vi "main.vi"() -> ()   [LabVIEW 2024]
uses:
  controls/#typedef_program_data_soundDB.ctl
  <vilib>/Utility/miscctls.llb/LVPoint32TypeDef.ctl
  controls/#typedef_program_states_soundDB.ctl
panel:
  out "error out":errorcluster
  in  "error in (no error)":errorcluster
  in  "Cluster":T1={"Sound intensity [dB]"=0, "Sound intensity: MIN"=0.0, "Sound intensity: MAX"=230.0, "Char array"=[], "Point32"={"Horizontal"=0, "Vertical"=0}, "drag?"=FALSE} {"Sound intensity [dB]" scale=0.0..100.0}
  out "To be moved":string
  in  "Sound intensity: MAX":dbl=230.0
  in  "Sound intensity: MIN":dbl
  out "Limit exceeded?":bool
  in  "Stop Button":bool
  in  "Sound intensity [dB]":u8(slide) scale=0.0..100.0
  # "85 dB"
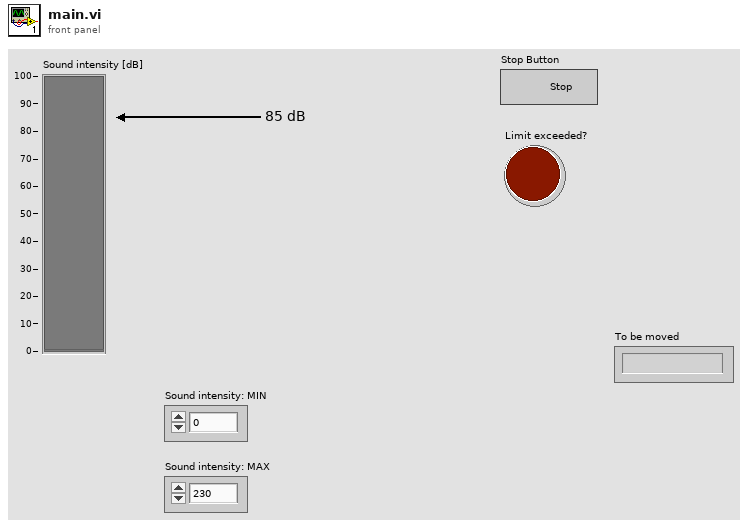
[diagram p1: front panel]
types:
  T1 = typedef "#typedef_program_data_soundDB.ctl" = cluster{"Sound intensity [dB]":u8, "Sound intensity: MIN":dbl, "Sound intensity: MAX":dbl, "Char array":i16[], "Point32":T2, "drag?":bool}
  T2 = typedef "LVPoint32TypeDef.ctl" = cluster{"Horizontal":i32, "Vertical":i32}
  T3 = typedef "#typedef_program_states_soundDB.ctl" = enum16{"application error", "init", "idle", "move", "Limit exceeded", "exit"}
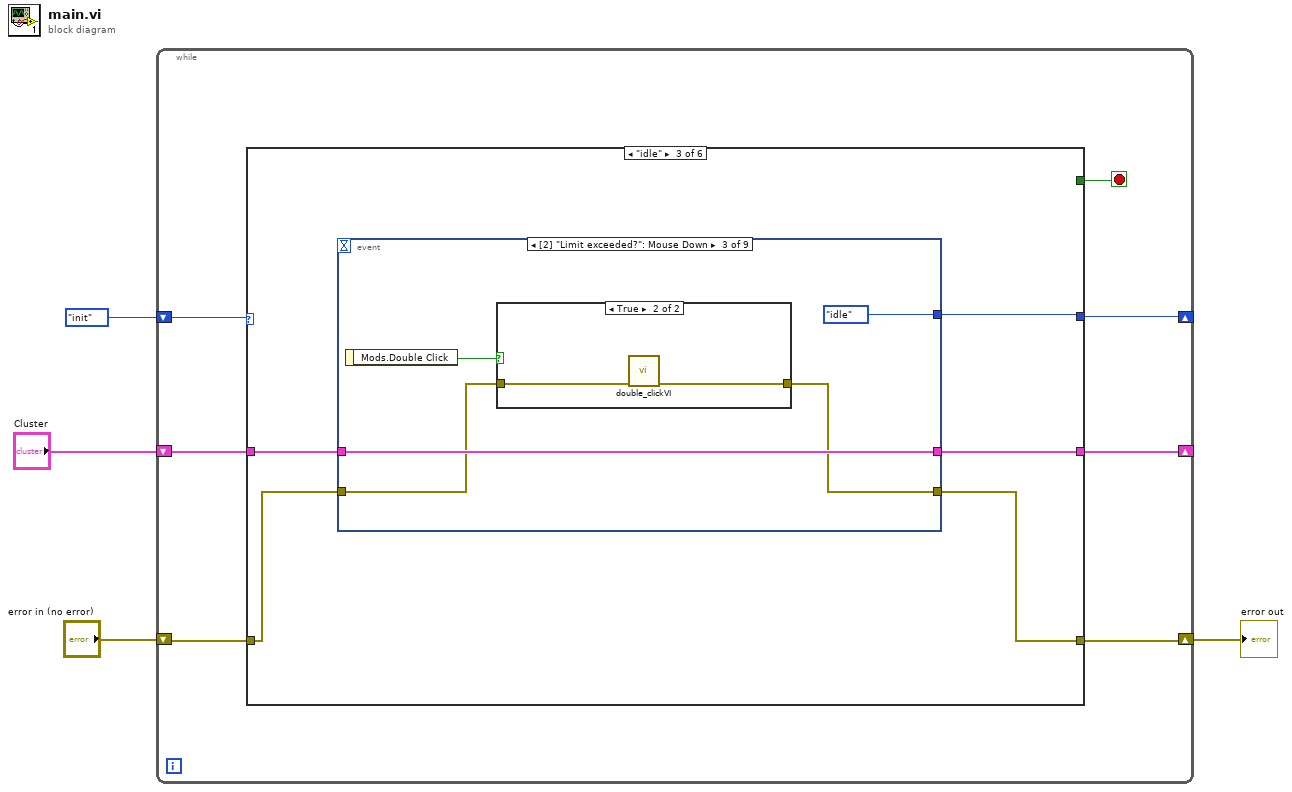
[diagram p0: block diagram]
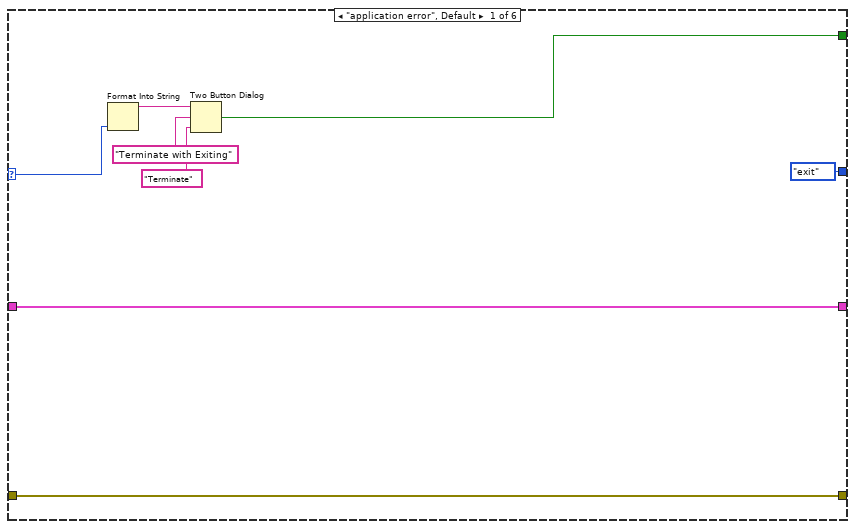
[diagram p2: hidden frame]
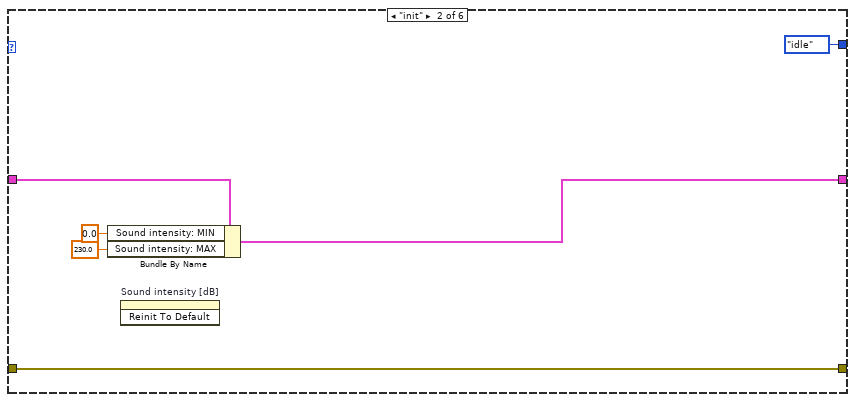
[diagram p3: hidden frame]
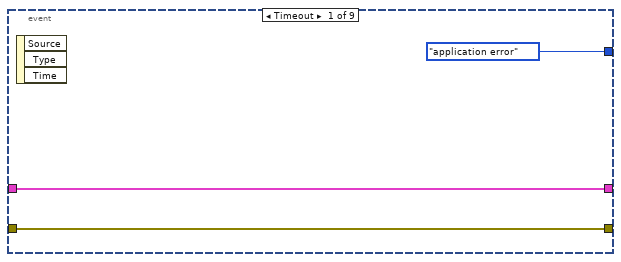
[diagram p4: hidden frame]
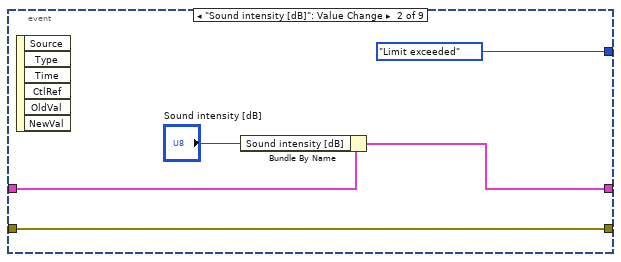
[diagram p5: hidden frame]
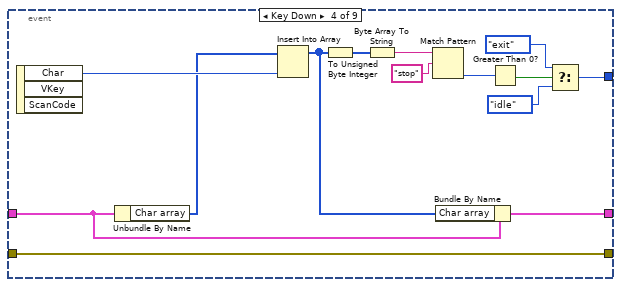
[diagram p7: hidden frame]
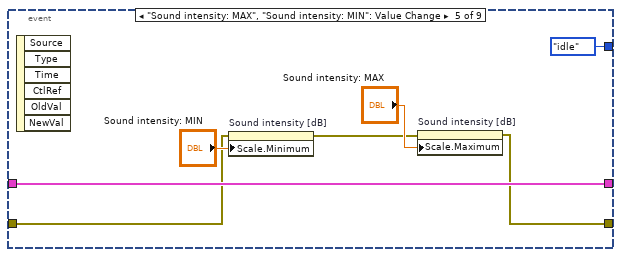
[diagram p8: hidden frame]
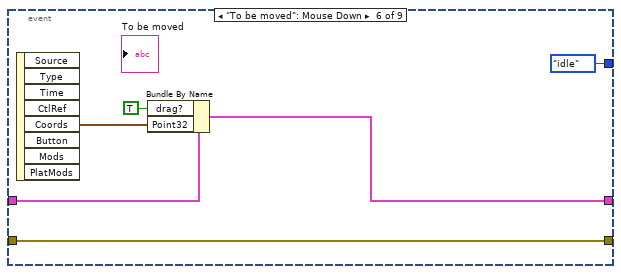
[diagram p9: hidden frame]
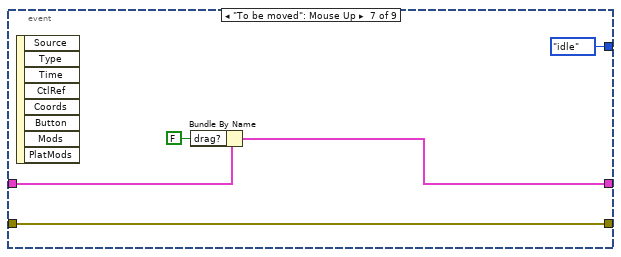
[diagram p10: hidden frame]
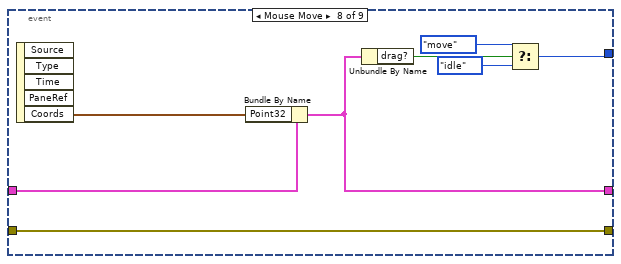
[diagram p11: hidden frame]
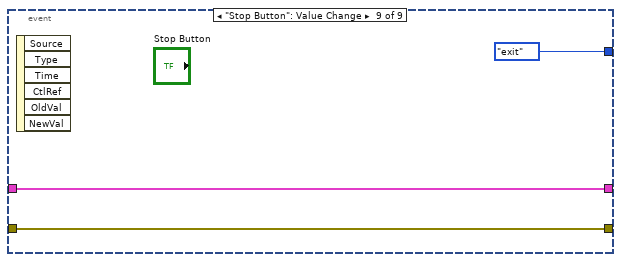
[diagram p12: hidden frame]
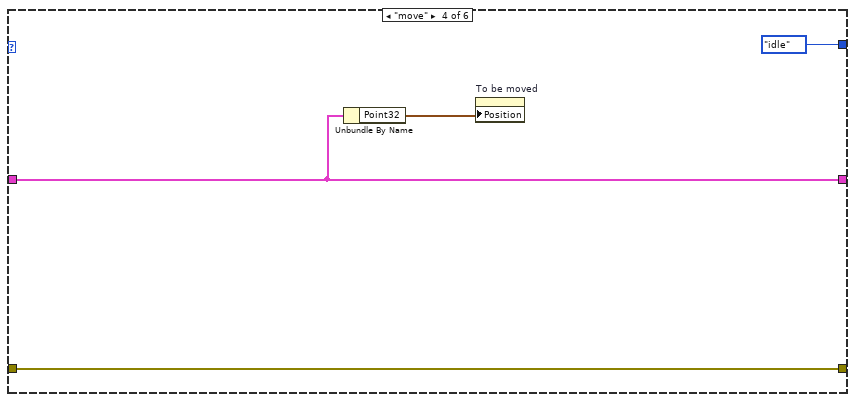
[diagram p13: hidden frame]
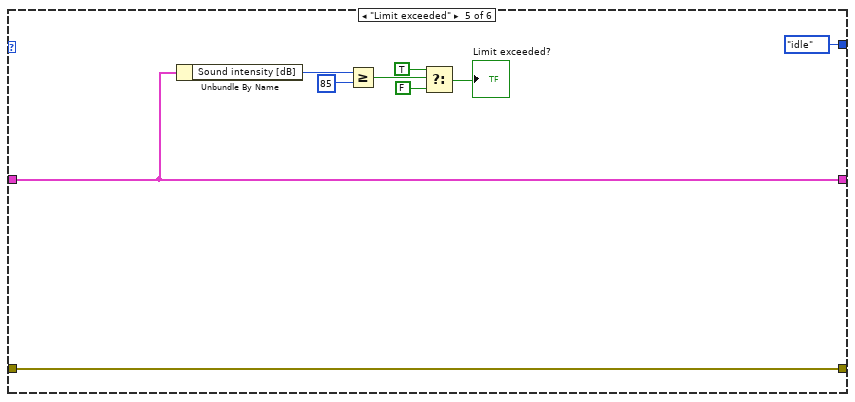
[diagram p14: hidden frame]
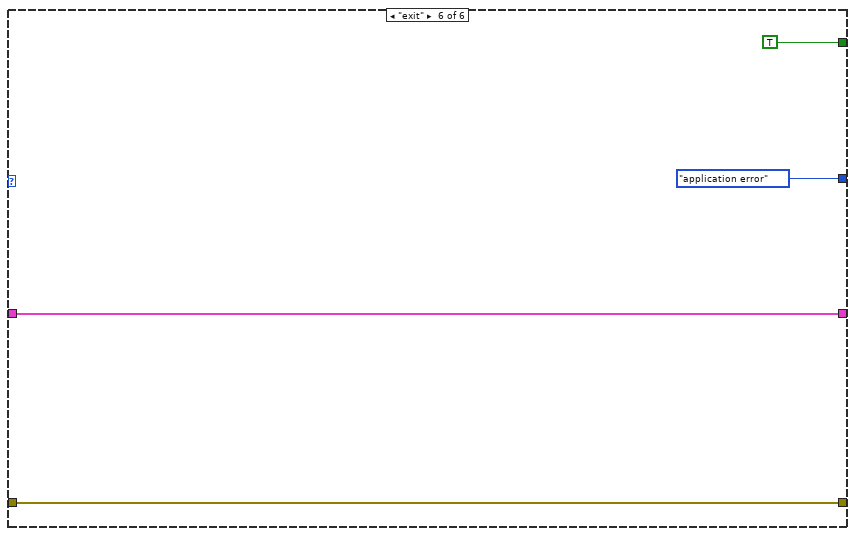
[diagram p15: hidden frame]
diagram:
  n1 = while {
    shift-right: [w9] -> _
    shift-left: #typedef_program_states_soundDB."init" ("Program States") -> [w11]
    shift-right: [w7] -> _
    shift-left: "Cluster" -> [w8]
    shift-right: [w5] -> w1
    shift-left: "error in (no error)" -> [w6]
    stop <- w10 stop-if-true
    n2 = case shown="\"idle\"" w11 {
      selector: w11 -> [w19 _ _ _ _ _]
      tunnel: [w15 _ _ _ _ TRUE] -> w10
      tunnel: [#typedef_program_states_soundDB."exit" ("Program States") #typedef_program_states_soundDB."idle" ("Program States") w30 #typedef_program_states_soundDB."idle" ("Program States") #typedef_program_states_soundDB."idle" ("Program States") #typedef_program_states_soundDB."application error" ("Program States")] -> w9
      tunnel: w8 -> [w13 w24 w29 w92 w96 w104]
      tunnel: [w13 w21 w28 w92 w96 w104] -> w7
      tunnel: w6 -> [w12 w20 w27 w90 w94 w103]
      tunnel: [w12 w20 w26 w90 w94 w103] -> w5
      frame "application error", Default {
        n3 = Format Into String(w19) -> (resulting string=w18:string)  [unwired: 3 in, 1 out]
        n4 = Two Button Dialog(message=w18, 1:"Terminate" ("F button name (\"Cancel\")"), 2:"Terminate with Exiting" ("T button name (\"OK\")")) -> (T button?=w15:bool)
      }
      frame "init" {
        n5 = Bundle By Name(cluster=w24, "Sound intensity: MIN"=0.0, "Sound intensity: MAX"=230.0) -> (w21:T1)
        n6 = invoke on="Sound intensity [dB]" class="Slide (strict)" method="Reinit To Default"() -> ()  [unwired: 3 in, 3 out]
      }
      frame "idle" {
        n7 = event shown="[2] \"Limit exceeded?\": Mouse Down" {
          selector: _ -> [_ _ _ _ _ _ _ _ _]
          dyn-events: _ -> [_ _ _ _ _ _ _ _ _]
          timeout: _ -> [_ _ _ _ _ _ _ _ _]
          tunnel: [#typedef_program_states_soundDB."application error" ("Program States") #typedef_program_states_soundDB."Limit exceeded" ("Program States") #typedef_program_states_soundDB."idle" ("Program States") w49 #typedef_program_states_soundDB."idle" ("Program States") #typedef_program_states_soundDB."idle" ("Program States") #typedef_program_states_soundDB."idle" ("Program States") w83 #typedef_program_states_soundDB."exit" ("Program States")] -> w30
          tunnel: w29 -> [w32 w36 w41 w58 w64 w72 w78 w82 w88]
          tunnel: [w32 w35 w41 w59 w64 w71 w76 w80 w88] -> w28
          tunnel: w27 -> [w31 w34 w40 w47 w63 w68 w74 w79 w87]
          tunnel: [w31 w34 w39 w47 w61 w68 w74 w79 w87] -> w26
          event Timeout {
            n8 = event-data() -> ()  [unwired: 1 in, 3 out]
          }
          event "Sound intensity [dB]": Value Change {
            n9 = event-data() -> ()  [unwired: 1 in, 6 out]
            n10 = Bundle By Name(cluster=w36, "Sound intensity [dB]"="Sound intensity [dB]") -> (w35:T1)
          }
          event "Limit exceeded?": Mouse Down {
            n11 = event-data() -> ("Mods.Double Click"=w43:bool)  [unwired: 1 in]
            n12 = case shown="True" w43 {
              tunnel: w40 -> [w44 w46]
              tunnel: [w44 w45] -> w39
              frame False {
              }
              frame True {
                n13 = call "double_clickVI.vi"("error in (no error)"=w46) -> ("error out"=w45:errorcluster)  [unwired: 10 in]
              }
            }
          }
          event Key Down {
            n14 = event-data() -> ("Char"=w60:i16)  [unwired: 1 in, 2 out]
            n15 = Unbundle By Name(w58) -> ("Char array"=w57:i16[])
            n16 = Insert Into Array(array=w57, new element=w60) -> (w55:i16[])  [unwired: 1 in]
            n17 = To Unsigned Byte Integer(number=w55) -> (unsigned 8bit integer=w56:u8[])
            n18 = Byte Array To String(unsigned byte array=w56) -> (string=w54:string)
            n19 = Match Pattern(string=w54, regular expression="stop") -> (offset past match=w52:i32)  [unwired: 1 in, 3 out]
            n20 = Bundle By Name(cluster=w58, "Char array"=w55) -> (w59:T1)
            n21 = Greater Than 0?(x=w52) -> (x > 0?=w51:bool)
            n22 = Select(t=#typedef_program_states_soundDB."exit" ("Program States"), s=w51, f=#typedef_program_states_soundDB."idle") -> (s? t:f=w49:T3)
          }
          event "Sound intensity: MAX", "Sound intensity: MIN": Value Change {
            n23 = event-data() -> ()  [unwired: 1 in, 6 out]
            n24 = property on="Sound intensity [dB]" class="Slide (strict)"(error in=w63, "Scale.Minimum"="Sound intensity: MIN") -> (error out=w62:errorcluster)  [unwired: 1 in, 1 out]
            n25 = property on="Sound intensity [dB]" class="Slide (strict)"(error in=w62, "Scale.Maximum"="Sound intensity: MAX") -> (error out=w61:errorcluster)  [unwired: 1 in, 1 out]
          }
          event "To be moved": Mouse Down {
            n26 = event-data() -> ("Coords"=w69:T2)  [unwired: 1 in, 7 out]
            n27 = Bundle By Name(cluster=w72, "drag?"=TRUE, "Point32"=w69) -> (w71:T1)
          }
          event "To be moved": Mouse Up {
            n28 = event-data() -> ()  [unwired: 1 in, 8 out]
            n29 = Bundle By Name(cluster=w78, "drag?"=FALSE) -> (w76:T1)
          }
          event Mouse Move {
            n30 = event-data() -> ("Coords"=w81:T2)  [unwired: 1 in, 4 out]
            n31 = Bundle By Name(cluster=w82, "Point32"=w81) -> (w80:T1)
            n32 = Unbundle By Name(w80) -> ("drag?"=w86:bool)
            n33 = Select(t=#typedef_program_states_soundDB."move" ("Program States"), s=w86, f=#typedef_program_states_soundDB."idle" ("Program States")) -> (s? t:f=w83:T3)
          }
          event "Stop Button": Value Change {
            n34 = event-data() -> ()  [unwired: 1 in, 6 out]
          }
        }
      }
      frame "move" {
        n35 = Unbundle By Name(w92) -> ("Point32"=w93:T2)
        n36 = property on="To be moved" class="Str"("Position"=w93) -> ()  [unwired: 2 in, 2 out]
      }
      frame "Limit exceeded" {
        n37 = Unbundle By Name(w96) -> ("Sound intensity [dB]"=w95:u8)
        n38 = Greater Or Equal?(x=w95, y=u8 85) -> (x >= y?=w102:bool)
        n39 = Select(t=TRUE, s=w102, f=FALSE) -> (s? t:f=→"Limit exceeded?":bool)
      }
      frame "exit" {
      }
    }
  }
  "error out" <- w1
